vi "Write Parameter to Word.vi"(8 "error in":errorcluster, 9 "parameter definition":T1={"start index"=10, "size"=19, "encoding"=enum."BNR", "signed"=FALSE, "scale multiplier"=1.0, "scale offset"=0.0}, 10 "data":dbl, 11 "32-bit Word in":refnum<class "32-bit Word.lvclass">) -> (0 "error out":errorcluster, 3 "32-bit Word out":refnum<class "32-bit Word.lvclass">)   [LabVIEW 2020, in "32-bit Word.lvclass"]
uses:
  32-bit Word.lvclass
  Parameter Definition.ctl
  <vilib>/NI/NI VeriStand Encoding and Decoding/Encoding.ctl
  ARINC 429.lvclass
  <vilib>/NI/NI VeriStand Encoding and Decoding/Encoding and Decoding.lvlib
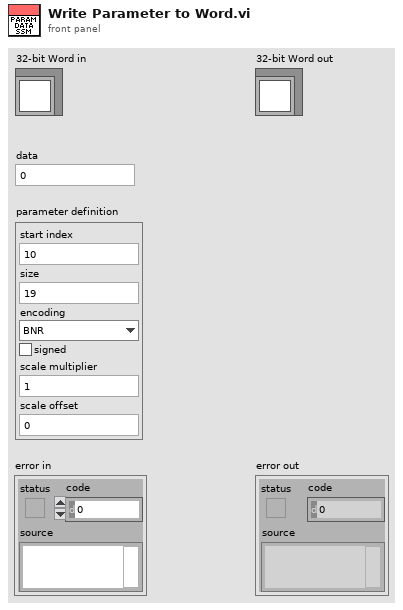
[diagram p1: front panel]
types:
  T1 = typedef "ARINC 429.lvclass/Parameter Definition.ctl" = cluster{"start index":i32, "size":i32, "encoding":T2, "signed":bool, "scale multiplier":dbl, "scale offset":dbl}
  T2 = typedef "Encoding and Decoding.lvlib/Encoding.ctl" = enum16{"BNR", "BCD", "Discrete"}
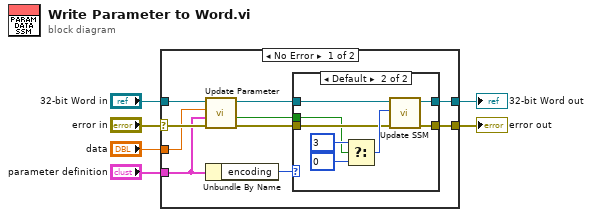
[diagram p0: block diagram]
diagram:
  n1 = case shown="No Error" "error in" {
    selector: "error in" -> [w13 w27]
    tunnel: "32-bit Word in" -> [w16 w28]
    tunnel: [w15 w28] -> w5
    tunnel: [w11 w27] -> w3
    tunnel: "data" -> [w10 _]
    tunnel: "parameter definition" -> [w9 _]
    frame No Error {
      n2 = call "Update Parameter.vi"("error in"=w13, "parameter definition"=w9, "data"=w10, "32-bit Word in"=w16) -> ("error out"=w12:errorcluster, "signed?"=w7:bool, "32-bit Word out"=w14:refnum<class "32-bit Word.lvclass">)  [unwired: 5 in]
      n3 = Unbundle By Name(w9) -> ("encoding"=w8:T2)
      n4 = case shown="Default" w8 {
        tunnel: [w18 w26] -> w15
        tunnel: w14 -> [w18 w22]
        tunnel: w12 -> [w17 w21]
        tunnel: [w17 w20] -> w11
        tunnel: w7 -> [_ w19]
        frame "Discrete" {
        }
        frame Default {
          n5 = Select(t=u8 3 ("SDI value"), s=w19, f=u8 0 ("SDI value")) -> (s? t:f=w23:u8)
          n6 = call-dynamic "Update SSM.vi"("error in"=w21, "SSM value"=w23, "32-bit Word in"=w22) -> ("error out"=w20:errorcluster, "32-bit Word out"=w26:refnum<class "32-bit Word.lvclass">)  [unwired: 7 in]
        }
      }
    }
    frame Error {
    }
  }
  "error out" <- w3
  "32-bit Word out" <- w5
